vi "readClassName.vi"(8 "error in (no error)":errorcluster, 11 "state in":refnum<class "state.lvclass">) -> (0 "error out":errorcluster, 2 "state name":string, 3 "state out":refnum<class "state.lvclass">)   [LabVIEW 2020, in "eos.lvlib" / "state.lvclass"]
uses:
  state.lvclass
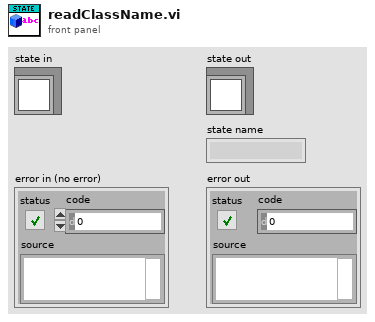
[diagram p1: front panel]
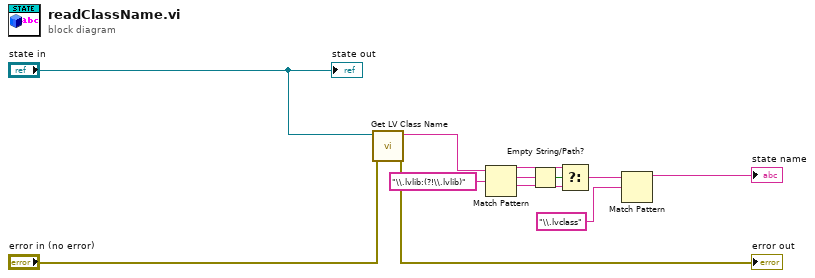
[diagram p0: block diagram]
diagram:
  n1 = call <vilib>:"Get LV Class Name.vi"("error in (no error)"="error in (no error)", "object"="state in") -> ("error out"=→"error out":errorcluster, "class name"=w4:string)  [unwired: 8 in]
  n2 = Match Pattern(string=w4, regular expression="\\.lvlib:(?!\\.lvlib)") -> (before substring=w6:string, match substring=w9:string, after substring=w7:string)  [unwired: 1 in, 1 out]
  n3 = Empty String/Path?(string/path=w9) -> (empty?=w8:bool)
  n4 = Select(t=w6, s=w8, f=w7) -> (s? t:f=w10:string)
  n5 = Match Pattern(string=w10, regular expression="\\.lvclass") -> (before substring=→"state name":string)  [unwired: 1 in, 3 out]
  "state out" <- "state in"
